vi "GetActualDepsListPath.vi"() -> (3 "Path":path)   [LabVIEW 2023, in "Reusables.lvlib"]
uses:
  Reusables.lvlib
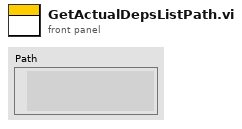
[diagram p1: front panel]
types:
  T1 = typedef "Reusables.lvlib/CICDPathConfigs.ctl" = cluster{"GlobalIncludePaths":path[], "GlobalExcludePaths":path[], "BuildSpecsIncludePaths":path[], "ActualDepsIncludePaths":path[], "WorkspacePath":path, "SourceFolderPaths":path[]}
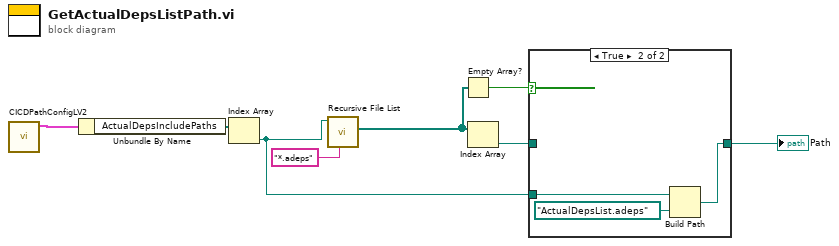
[diagram p0: block diagram]
diagram:
  n1 = call "CICDPathConfigLV2.vi"() -> ("CICD Path Config Out"=w6:T1)  [unwired: 11 in]
  n2 = Unbundle By Name(w6) -> ("ActualDepsIncludePaths"=w7:path[])
  n3 = Index Array(array=w7) -> (element=w3:path)  [unwired: 1 in]
  n4 = call <vilib>:"Recursive File List.vi"("pattern"="*.adeps", "Folder Path"=w3) -> ("All Files in Dir"=w5:path[])  [unwired: 5 in, 4 out]
  n5 = Empty Array?(array=w5) -> (empty?=w4:bool)
  n6 = Index Array(array=w5) -> (element=w2:path)  [unwired: 1 in]
  n7 = case shown="True" w4 {
    tunnel: w3 -> [_ w12]
    tunnel: w2 -> [w9 _]
    tunnel: [w9 w10] -> w1
    frame False {
    }
    frame True {
      n8 = Build Path(base path=w12, name or relative path=path "ActualDepsList.adeps") -> (appended path=w10:path)
    }
  }
  "Path" <- w1
